vi "jMsg_SnakeProcessor_ConfigureBoard (create).vi"(8 "error in (no error)":errorcluster, 10 "Height":i32, 11 "Width":i32) -> (0 "error out":errorcluster, 3 "jMsg_SnakeProcessor_ConfigureBoard":refnum<class "jMsg_SnakeProcessor_ConfigureBoard.lvclass">)   [LabVIEW 2019, in "jMsg_SnakeProcessor_ConfigureBoard.lvclass"]
doc: "This VI is used to create the jMsg\n\n\nJSMA Message Wizard 0.2.0.5\nRob Humfeld - Jet Engineering\nCopyright (c) 2020, Jet Engineering"
uses:
  jMsg_SnakeProcessor_ConfigureBoard.lvclass
  C:/Program Files/National Instruments/LabVIEW 2019/user.lib/Jet Engineering/JSMA/Libraries/jMsg Class/jMsg.lvclass
  <userlib>/Jet Engineering/JSMA/Libraries/jMsg Class/jMsg.lvclass/jMsg.ctl
  jMsg_SnakeProcessor_ConfigureBoard.lvclass/jMsg_SnakeProcessor_ConfigureBoard.ctl
  <userlib>/Jet Engineering/JSMA/Libraries/Shared/JSMA_GetClassName.vi
  <vilib>/Utility/LVClass/Get LV Class Path.vi
  <userlib>/Jet Engineering/JSMA/Libraries/jMsg Class/jMsg.lvclass
panel:
  in  "jMsg_SnakeProcessor_ConfigureBoard":refnum<class "jMsg_SnakeProcessor_ConfigureBoard.lvclass">
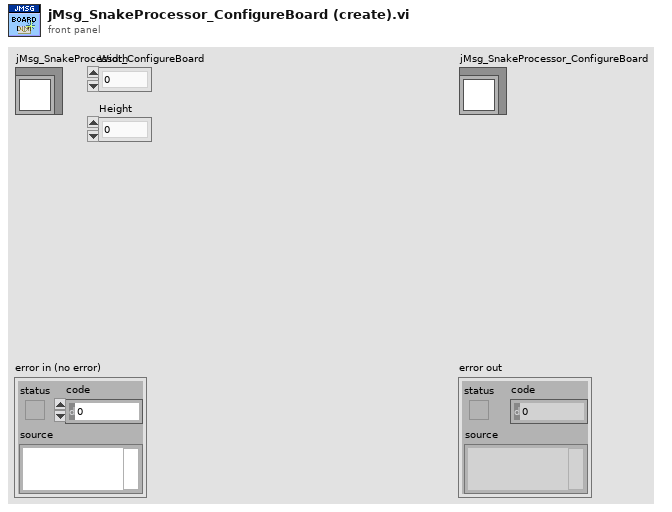
[diagram p1: front panel]
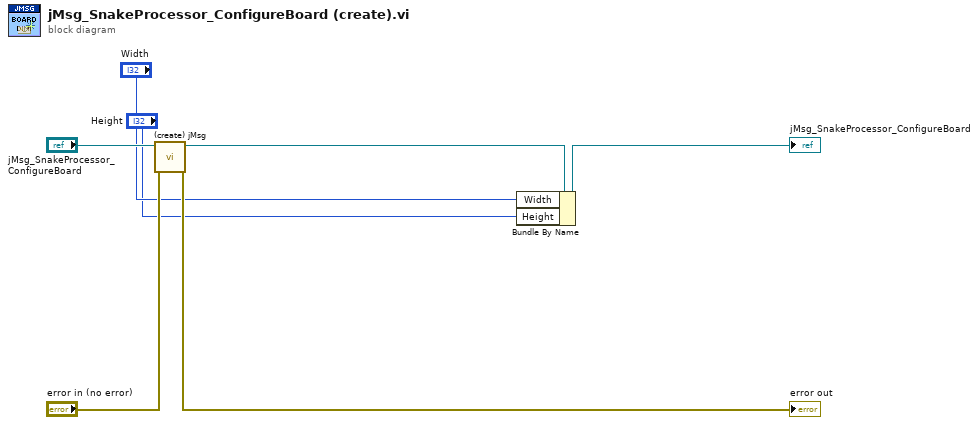
[diagram p0: block diagram]
diagram:
  n1 = call <userlib>:"(create) jMsg.vi"("error in (no error)"="error in (no error)", "jMsg in"="jMsg_SnakeProcessor_ConfigureBoard") -> ("error out"=→"error out":errorcluster, "jMsg out"=w3:refnum<class "jMsg_SnakeProcessor_ConfigureBoard.lvclass">)  [unwired: 8 in]
  n2 = Bundle By Name(cluster=w3, "Width"="Width", "Height"="Height") -> (→"jMsg_SnakeProcessor_ConfigureBoard":refnum<class "jMsg_SnakeProcessor_ConfigureBoard.lvclass">)
